vi "fileHead.vi"(0 "df":dbl=0.1, 1 "f_min":dbl=24.0, 3 "f_max":dbl=30.0, 4 "k_num":dbl=31.0, 5 "x_max":dbl=200.0, 6 "dx":dbl=5.0, 7 "x_min":dbl, 8 "distance":dbl=150.0, 9 "stepper_type":dbl) -> (2 "输出":string)   [LabVIEW 2018]
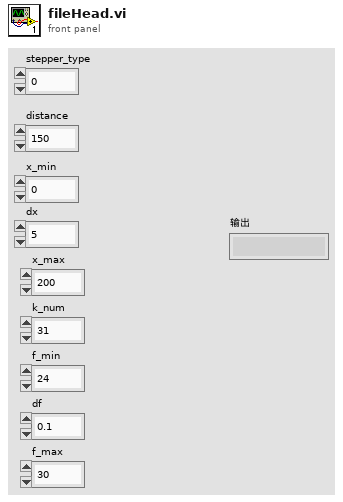
[diagram p1: front panel]
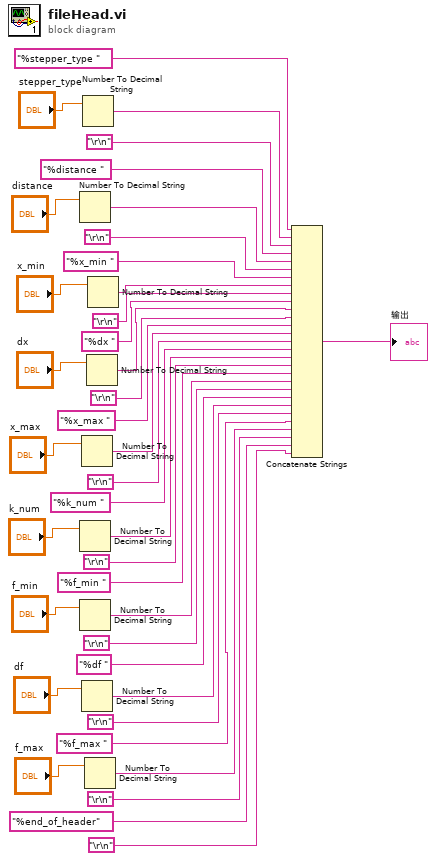
[diagram p0: block diagram]
diagram:
  n1 = Number To Decimal String(number="distance") -> (decimal integer string=w26:string)  [unwired: 1 in]
  n2 = Number To Decimal String(number="k_num") -> (decimal integer string=w14:string)  [unwired: 1 in]
  n3 = Number To Decimal String(number="f_min") -> (decimal integer string=w11:string)  [unwired: 1 in]
  n4 = Number To Decimal String(number="x_max") -> (decimal integer string=w17:string)  [unwired: 1 in]
  n5 = Number To Decimal String(number="df") -> (decimal integer string=w8:string)  [unwired: 1 in]
  n6 = Number To Decimal String(number="stepper_type") -> (decimal integer string=w29:string)  [unwired: 1 in]
  n7 = Number To Decimal String(number="f_max") -> (decimal integer string=w5:string)  [unwired: 1 in]
  n8 = Number To Decimal String(number="dx") -> (decimal integer string=w20:string)  [unwired: 1 in]
  n9 = Number To Decimal String(number="x_min") -> (decimal integer string=w23:string)  [unwired: 1 in]
  n10 = Concatenate Strings("%stepper_type ", w29, "\r\n", "%distance ", w26, "\r\n", "%x_min ", w23, "\r\n", "%dx ", w20, "\r\n", "%x_max ", w17, "\r\n", "%k_num ", w14, "\r\n", "%f_min ", w11, "\r\n", "%df ", w8, "\r\n", "%f_max ", w5, "\r\n", "%end_of_header", "\r\n") -> (→"输出":string)
